vi "ClawSetpointIndex.vi"(10 "On Bert?":bool=TRUE, 11 "Claw States":T1) -> (3 "Setpoint":dbl)   [LabVIEW 2014]
uses:
  Typedefs/ClawStates.ctl
panel:
  in  "Ernie Claw LUT":dbl[](array[numeric])=[0.0, 0.88, 0.48, 0.57, 0.65]
  in  "Bert Claw LUT":dbl[](array[numeric])=[0.0, 0.47, 0.11, 0.24, 0.32]
  # "Manual"
  # "Claw Open"
  # "Claw Closed"
  # "Claw Slight Open"
  # "Flip Can"
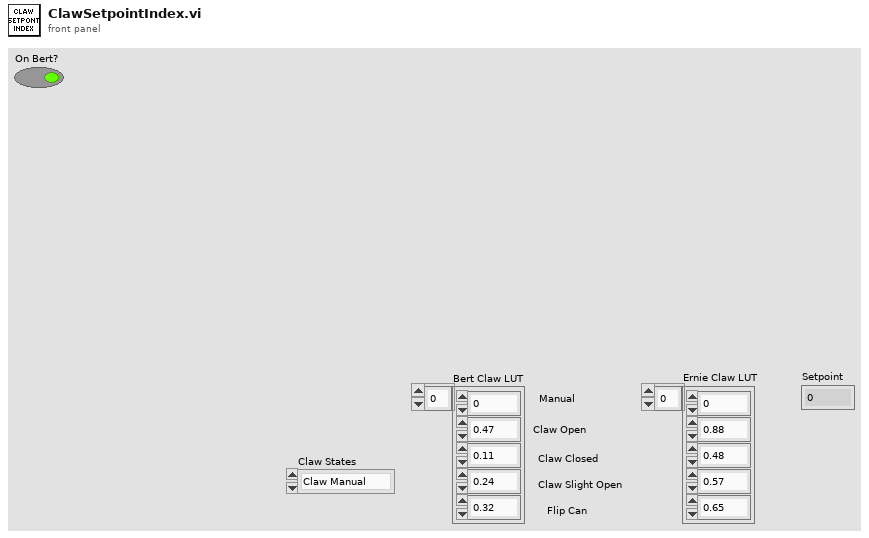
[diagram p1: front panel]
types:
  T1 = typedef "ClawStates.ctl" = enum16{"Claw Manual ", "Claw Open", "Claw Closed", "Claw Slight Open", "Flip Can"}
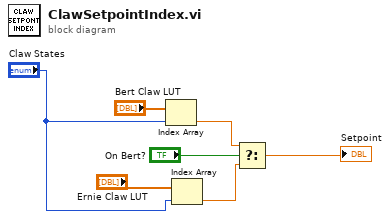
[diagram p0: block diagram]
diagram:
  n1 = Index Array(array="Bert Claw LUT", index="Claw States") -> (element=w4:dbl)
  n2 = Index Array(array="Ernie Claw LUT", index="Claw States") -> (element=w3:dbl)
  n3 = Select(t=w4, s="On Bert?", f=w3) -> (s? t:f=→"Setpoint":dbl)
